vi "Analog Read.vi"(7 "Analog Ref Override":dbl, 8 "Error In":errorcluster={"status"=TRUE, "code"=5001, "source"="LVH-LINX.lvlib:Generate Error.vi<ERR>\nA timeout occured while waiting for the LINX device to respond."}, 10 "AI Channels":u8[](array[numeric])=[0], 11 "LINX Device Config":T1={"Interface"=enum."Serial", "COM Port"="COM5", "TCP Configuration"={"IP Address"="", "Port"=0}, "Device Family"=enum."National Instruments", "Device ID"=0, "Device Name"="", "TCP Ref"=refnum}) -> (0 "Error Out":errorcluster={"status"=TRUE, "code"=5001, "source"="LVH-LINX.lvlib:Generate Error.vi<ERR>\nA timeout occured while waiting for the LINX device to respond."}, 1 "AI Ref":dbl, 2 "Voltages":dbl[](array[numeric]), 3 "LINX Device Config":T1={"Interface"=enum."Serial", "COM Port"="COM5", "TCP Configuration"={"IP Address"="", "Port"=0}, "Device Family"=enum."National Instruments", "Device ID"=0, "Device Name"="", "TCP Ref"=refnum})   [LabVIEW 2013, in "LVH-LINX.lvlib" / "Device.lvlib"]
uses:
  <vilib>/LabVIEW Hacker/LINX/Private/Device/Device.lvlib
  <vilib>/LabVIEW Hacker/LINX/Private/Device/Type Defs/LINX Device Config.ctl
  <vilib>/LabVIEW Hacker/LINX/Private/Type Defs/Interface.ctl
  <vilib>/LabVIEW Hacker/LINX/Private/Device/Type Defs/TCP Config.ctl
  <vilib>/LabVIEW Hacker/LINX/Private/Type Defs/Device Family.ctl
  <vilib>/LabVIEW Hacker/LINX/Private/Type Defs/Error Type.ctl
  <vilib>/LabVIEW Hacker/LINX/LVH-LINX.lvlib
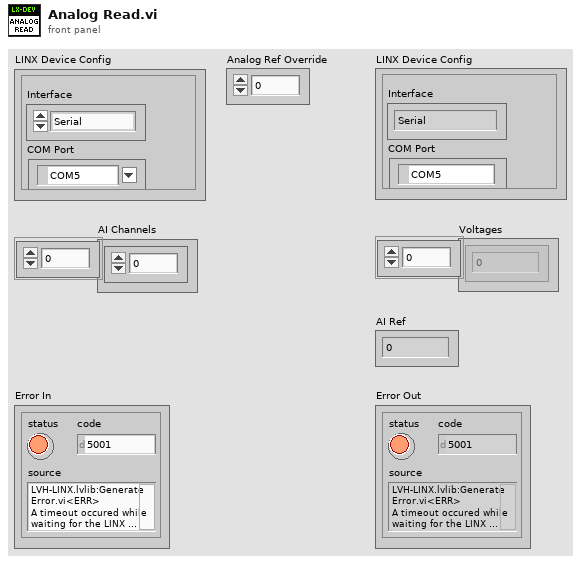
[diagram p1: front panel]
types:
  T1 = typedef "LVH-LINX.lvlib/Device.lvlib/LINX Device Config.ctl" = cluster{"Interface":T2, "COM Port":refnum<visa-resource-name>, "TCP Configuration":T3, "Device Family":T4, "Device ID":u8, "Device Name":string, "TCP Ref":refnum<k5>}
  T2 = typedef "LVH-LINX.lvlib/Interface.ctl" = enum16{"Serial", "TCP"}
  T3 = typedef "LVH-LINX.lvlib/Device.lvlib/TCP Config.ctl" = cluster{"IP Address":string, "Port":u16}
  T4 = typedef "LVH-LINX.lvlib/Device Family.ctl" = enum8{"National Instruments", "Digilent", "Arduino"}
  T5 = typedef "LVH-LINX.lvlib/Error Type.ctl" = enum16{"Unknown", "Timeout", "Corrupt Return Packet", "Unable To Connect", "Command Not Supported", "Channel DNE", "Invalid COM Config"}
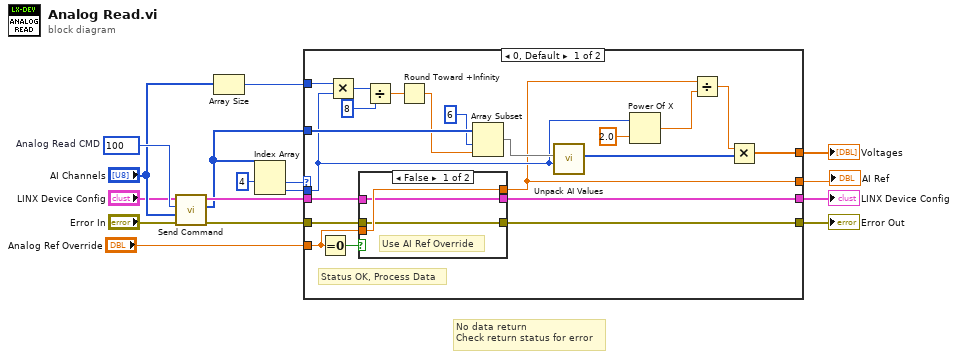
[diagram p0: block diagram]
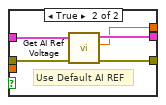
[diagram p2: hidden frame]
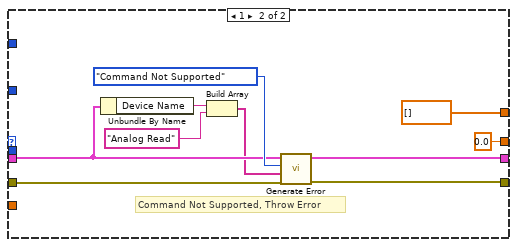
[diagram p3: hidden frame]
diagram:
  w15 = u16 100  # Analog Read CMD
  # "No data return\nCheck return status for error"
  n1 = call <vilib>:"Send Command.vi"("Error In"="Error In", "ARGS"="AI Channels", "CMD"=w15, "LINX Device Config"="LINX Device Config") -> ("Error Out"=w9:errorcluster, "Response"=w8:u8[], "LINX Device Config"=w11:T1)  [unwired: 4 in, 1 out]
  n2 = Array Size(array="AI Channels") -> (size(s)=w6:i32)
  n3 = Index Array(array=w8, index #1=4 ("index")) -> (element #1=w13:u8, element #2=w5:u8)  [unwired: 1 in]
  n4 = case shown="0, Default" w13 {
    tunnel: [w21 w53] -> w12
    tunnel: w11 -> [w22 w49]
    tunnel: [w19 w54] -> w10
    tunnel: w9 -> [w20 w55]
    tunnel: w8 -> [w37 _]
    tunnel: w6 -> [w36 _]
    tunnel: [w27 dbl[] []] -> w3
    tunnel: w5 -> [w25 _]
    tunnel: "Analog Ref Override" -> [w18 _]
    tunnel: [w17 0.0 ("AI Ref (V)")] -> w1
    frame 0, Default {
      # "Status OK, Process Data"
      n5 = Equal To 0?(x=w18) -> (x = 0?=w23:bool)
      n6 = Multiply(x=w36, y=w25) -> (x*y=w35:i32)
      n7 = case shown="False" w23 {
        tunnel: w22 -> [w39 w45]
        tunnel: [w39 w44] -> w21
        tunnel: w20 -> [w38 w43]
        tunnel: [w38 w42] -> w19
        tunnel: [w40 w41] -> w17
        tunnel: w18 -> [w40 _]
        frame False {
          # "Use AI Ref Override"
        }
        frame True {
          # "Use Default AI REF"
          n8 = call <vilib>:"Get AI Ref Voltage.vi"("Error In"=w43, "LINX Device Config"=w45) -> ("Error Out"=w42:errorcluster, "AI Ref (V)"=w41:dbl, "LINX Device Config"=w44:T1)  [unwired: 7 in]
        }
      }
      n9 = Divide(x=w35, y=8) -> (x/y=w33:dbl)
      n10 = Round Toward +Infinity(x=w33) -> (ceil(x): smallest int >= x=w31:dbl)
      n11 = Array Subset(array=w37, index=6, length=w31) -> (w30:u8[])
      n12 = call <vilib>:"Unpack AI Values.vi"("Resolution"=w25, "Values"=w30) -> ("ADC Ticks"=w29:u32[])  [unwired: 9 in]
      n13 = Power Of X(1:2.0 ("x"), 2:w25) -> (0:w24:dbl)
      n14 = Divide(x=w17, y=w24) -> (x/y=w28:dbl)
      n15 = Multiply(x=w28, y=w29) -> (x*y=w27:dbl[])
    }
    frame 1 {
      # "Command Not Supported, Throw Error"
      n16 = Unbundle By Name(w49) -> ("Device Name"=w51:string)
      n17 = Build Array(w51, "Analog Read") -> (w48:string[])
      n18 = call <vilib>:"Generate Error.vi"("Error In"=w55, "Arguments"=w48, "Error Type"=Error_Type."Command Not Supported", "LINX Device Config"=w49) -> ("Error Out"=w54:errorcluster, "LINX Device Config"=w53:T1)  [unwired: 6 in]
    }
  }
  "Error Out" <- w10
  "LINX Device Config" <- w12
  "Voltages" <- w3
  "AI Ref" <- w1
